vi "Parse TOML String.vi"(8 "error in (no error)":errorcluster, 11 "String":string) -> (0 "error out":errorcluster, 3 "Value":T1)   [LabVIEW 2020, in "TOML.lvlib"]
uses:
  TOML.lvlib
  TOML Value.ctl
  Key-Value Pair.ctl
  Value.ctl
  Value Type.ctl
  State.ctl
  Context.ctl
  Table Context.ctl
  Table Array Context.ctl
  Array Context.ctl
  <vilib>/regexp/Match Regular Expression.xnode
  <vilib>/ErrorRing/Error Ring.xnode
  <vilib>/JDP Science/JDP Science Common Utilities/Timestamp/JDP Timestamp.lvlib
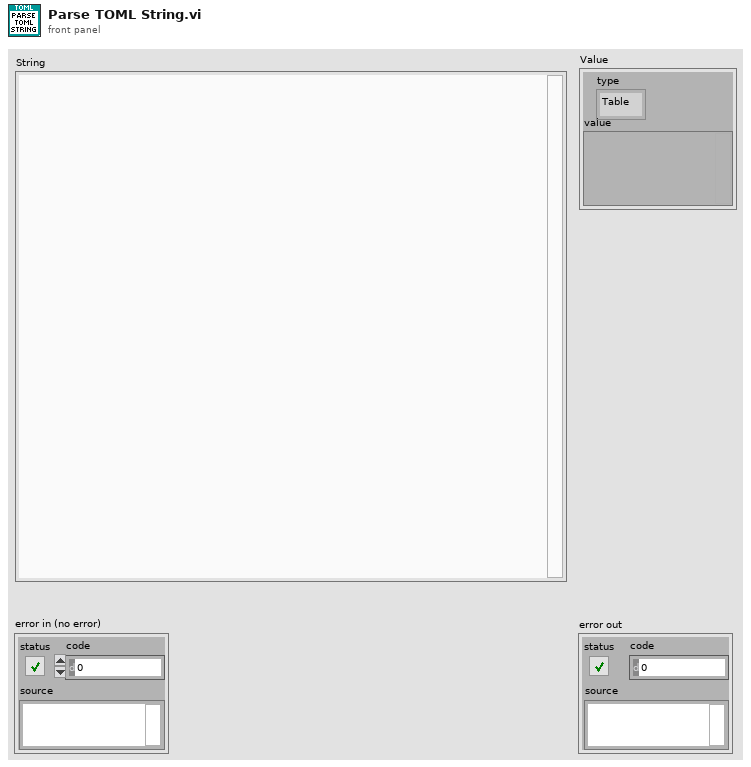
[diagram p1: front panel]
types:
  T1 = typedef "TOML.lvlib/TOML Value.ctl" = cluster{"type":enum16{"Table", "Array", "String", "Integer", "Float", "Boolean", "Offset Date-Time", "Local Date-Time", "Local Date", "Local Time", "Path"}, "value":variant}
  T2 = typedef "TOML.lvlib/Key-Value Pair.ctl" = cluster{"Key":string, "Value":T3}
  T3 = typedef "TOML.lvlib/Value.ctl" = cluster{"Type":T4, "Value":variant}
  T4 = typedef "TOML.lvlib/Value Type.ctl" = enum16{"Table", "Array", "String", "Integer", "Float", "Boolean", "Offset Date-Time", "Local Date-Time", "Local Date", "Local Time", "Path"}
  T5 = enum16{"Table", "Array", "String", "Integer", "Float", "Boolean", "Offset Date-Time", "Local Date-Time", "Local Date", "Local Time"}
  T6 = typedef "TOML.lvlib/Table Context.ctl" = cluster{"Table":T2[], "Key":string, "Defined Keys":string[]}
  T7 = typedef "TOML.lvlib/Context.ctl" = cluster{"Type":enum16{"Table", "Array", "Inline Table", "Table Array"}, "Value":variant}
  T8 = typedef "TOML.lvlib/State.ctl" = enum16{"Table", "Value", "Inline Table"}
  T9 = typedef "TOML.lvlib/Table Array Context.ctl" = cluster{"Table Array":cluster{"Table":T2[]}[], "Index":i32, "Key":string}
  T10 = typedef "TOML.lvlib/Array Context.ctl" = cluster{"Array":T3[], "Index":i32, "Empty":bool, "Type":T4}
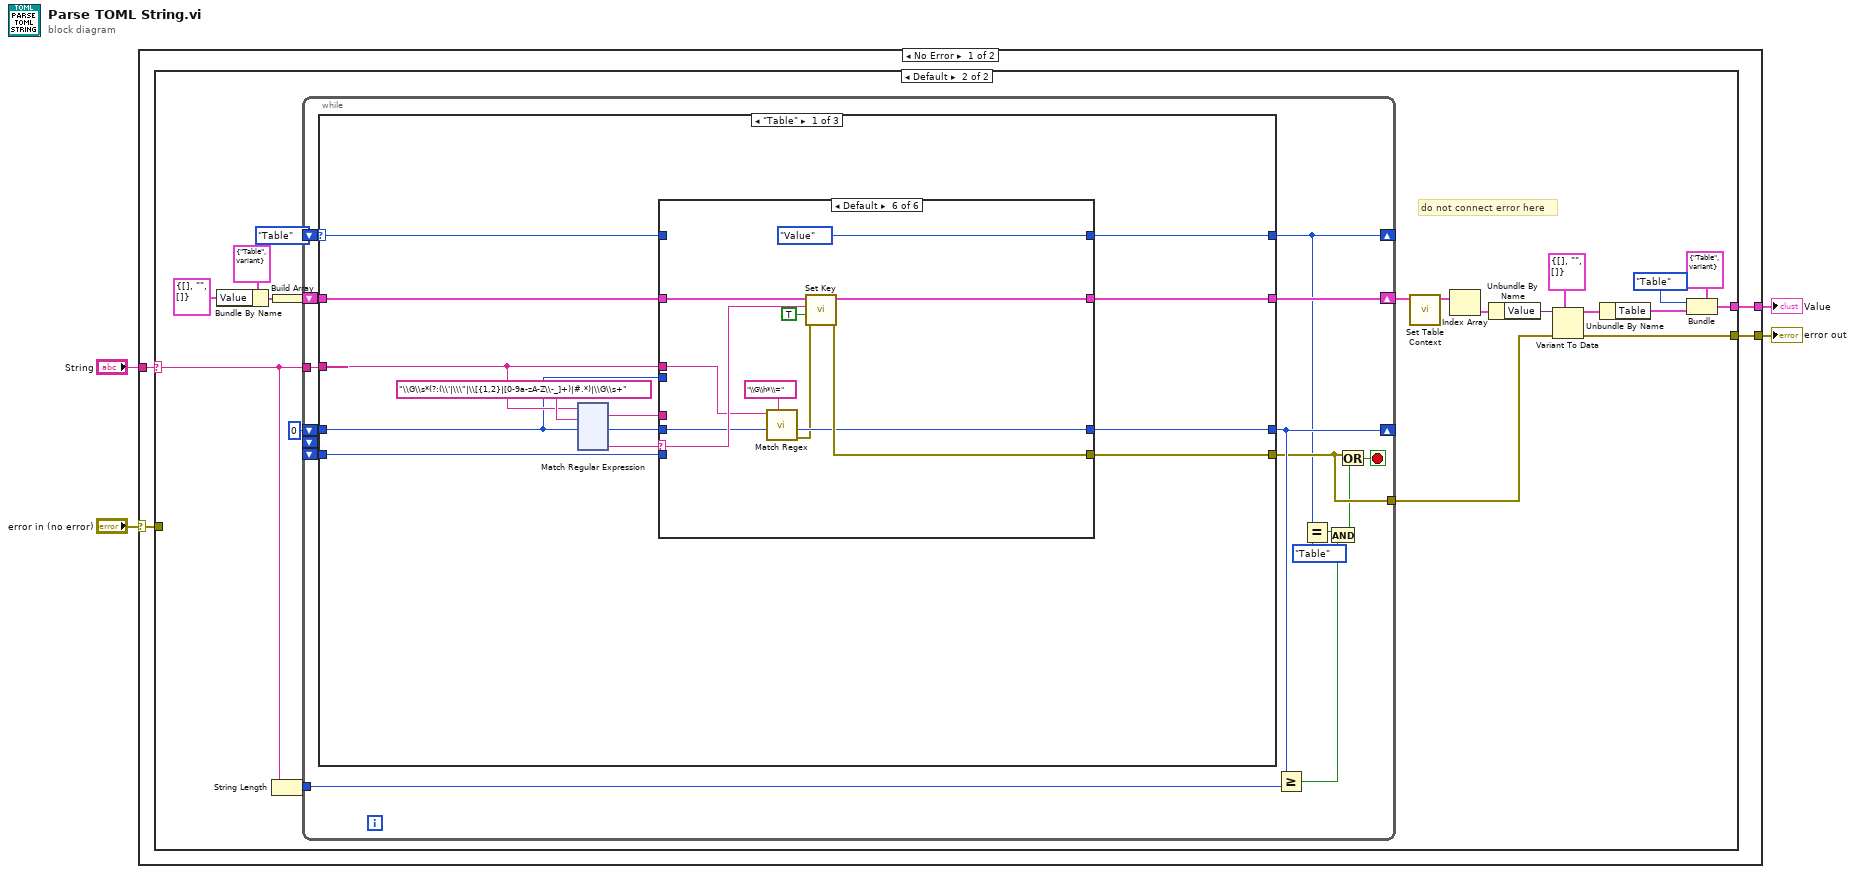
[diagram p0: block diagram]
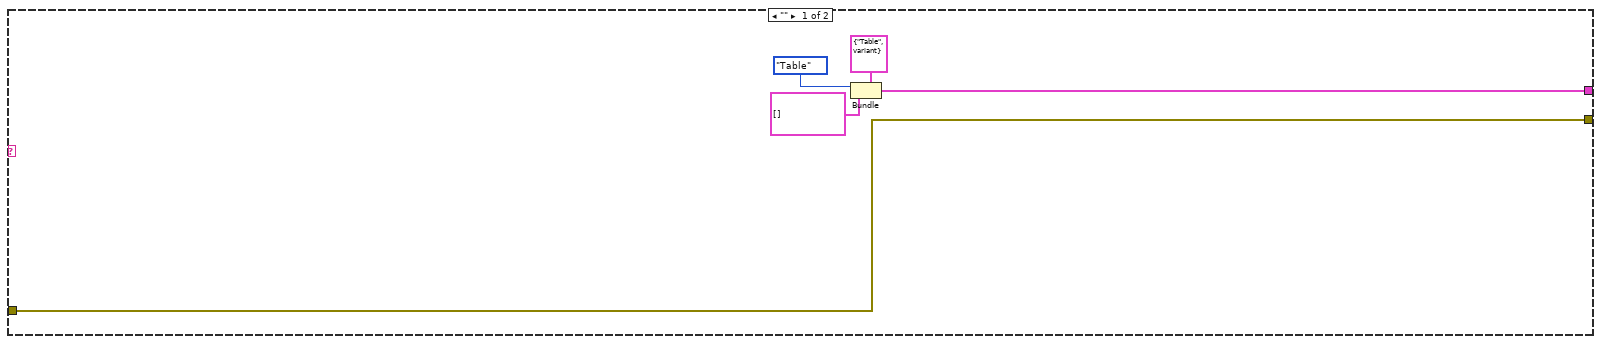
[diagram p2: hidden frame]
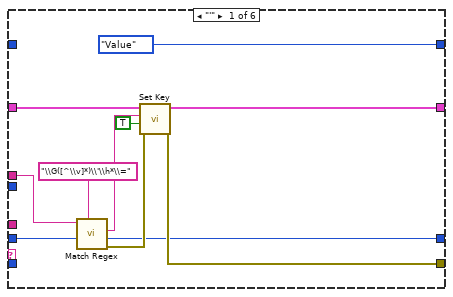
[diagram p3: hidden frame]
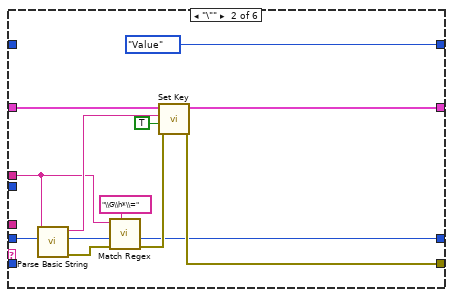
[diagram p4: hidden frame]
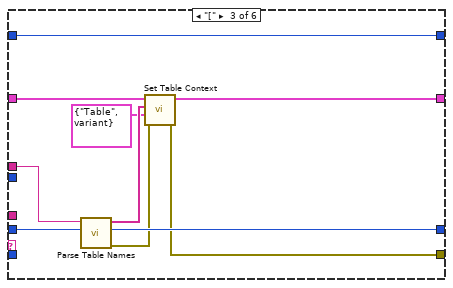
[diagram p5: hidden frame]
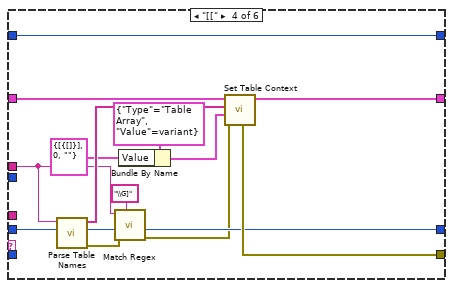
[diagram p6: hidden frame]
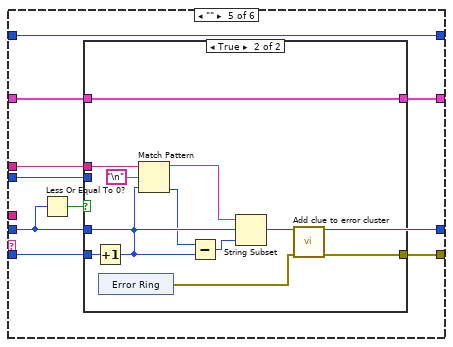
[diagram p7: hidden frame]
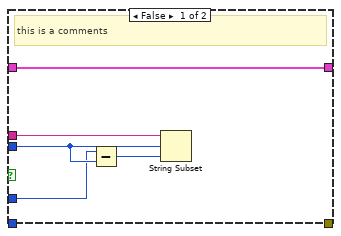
[diagram p8: hidden frame]
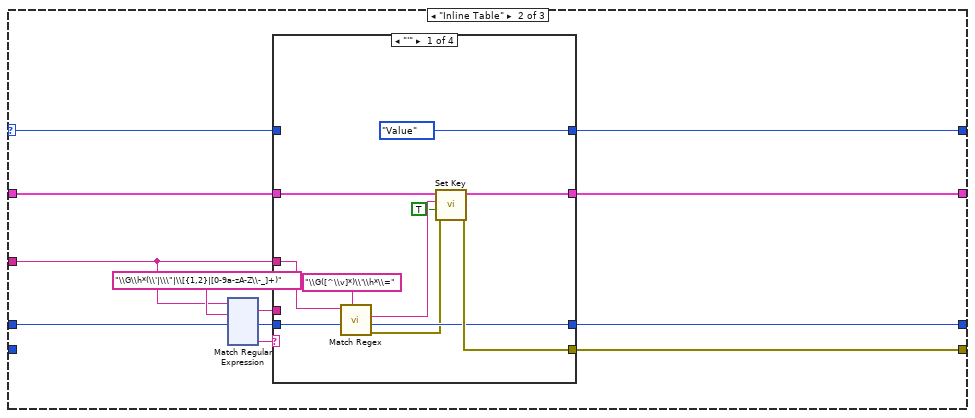
[diagram p9: hidden frame]
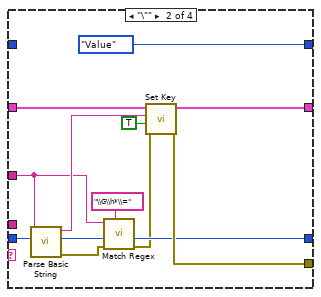
[diagram p10: hidden frame]
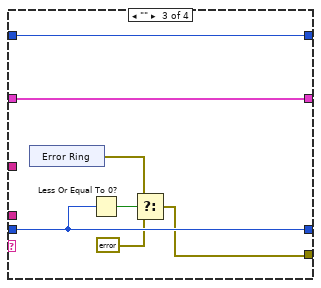
[diagram p11: hidden frame]
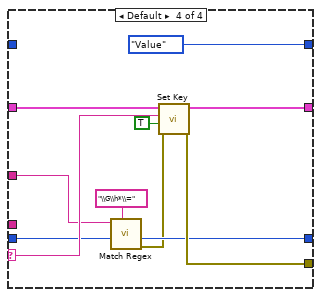
[diagram p12: hidden frame]
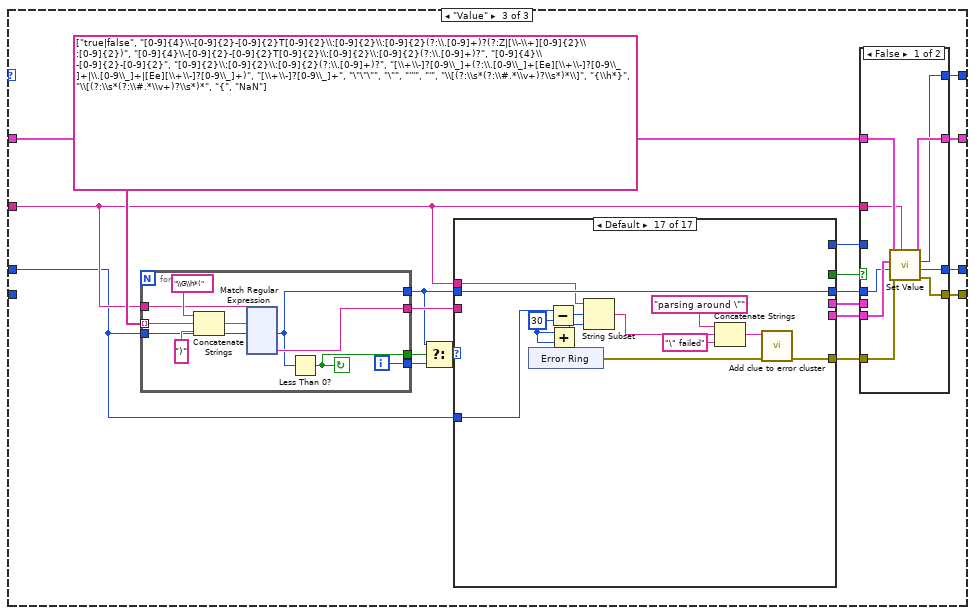
[diagram p13: hidden frame]
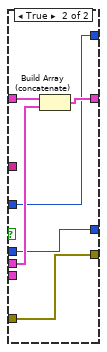
[diagram p14: hidden frame]
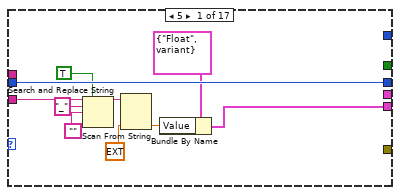
[diagram p15: hidden frame]
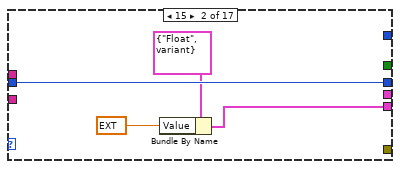
[diagram p16: hidden frame]
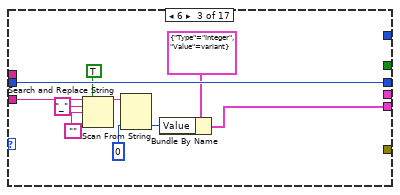
[diagram p17: hidden frame]
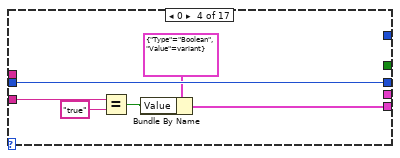
[diagram p18: hidden frame]
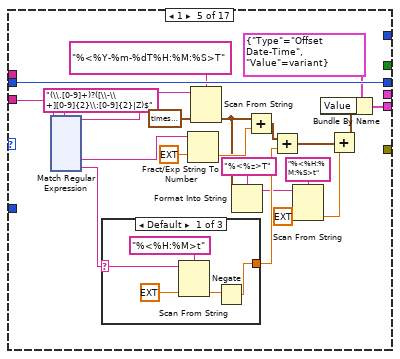
[diagram p19: hidden frame]
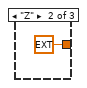
[diagram p20: hidden frame]
diagram:
  n1 = case shown="No Error" "error in (no error)" {
    selector: "error in (no error)" -> [w5 w846]
    tunnel: "String" -> [w8 _]
    tunnel: [w6 _] -> w1
    tunnel: [w7 w846] -> w3
    frame No Error {
      n2 = case shown="Default" w8 {
        selector: w8 -> [_ w32]
        tunnel: [w9 w24] -> w7
        tunnel: [w10 w20] -> w6
        tunnel: w5 -> [w9 _]
        frame "" {
          n3 = Bundle(cluster=T1 {"type"=enum."Table", "value"=variant} ("Value"), "type"=T5."Table" ("Type"), "value"=T2[] [] ("Table")) -> (w10:T1)
        }
        frame Default {
          w15 = 0
          # "do not connect error here"
          n4 = Bundle By Name(cluster=T7 {"Type"=enum."Table", "Value"=variant} ("Context"), "Value"=T6 {"Table"=[], "Key"="", "Defined Keys"=[]} ("Table Context")) -> (w17:T7)
          n5 = String Length(string=w32) -> (length=w31:i32)
          n6 = Build Array(w17) -> (w16:T7[])
          n7 = while {
            tunnel: w32 -> [w47]
            shift-right: [w37] -> _
            shift-left: State."Table" ("State") -> [w48]
            shift-right: [w45] -> w30
            shift-left: w16 -> [w44]
            shift-right: [w40] -> _
            shift-left: w15 -> [w46]
            tunnel: w31 -> [w42]
            tunnel: [w39] -> w14
            shift-left: w15 -> [_]
            shift-left: w15 -> [w34]
            stop <- w43 stop-if-true
            n8 = case shown="\"Table\"" w48 {
              selector: w48 -> [w57 w271 _]
              tunnel: w47 -> [w51 w265 w436]
              tunnel: w46 -> [w49 w264 w435]
              tunnel: [w58 w272 w440] -> w37
              tunnel: [w56 w270 w447] -> w45
              tunnel: w44 -> [w55 w269 w446]
              tunnel: [w59 w273 w437] -> w40
              tunnel: [w54 w268 w444] -> w39
              tunnel: w34 -> [w50 _ _]
              frame "Table" {
                n9 = xnode "Match Regular Expression"("input string"=w51, "regular expression"="\\G\\s*(?:(\\'|\\\"|\\[{1,2}|[0-9a-zA-Z\\-_]+)|#.*)|\\G\\s+", "offset (0)"=w49) -> ("whole match"=w52:string, "offset past match"=w60:i32, "submatch 1"=w53:string)  [unwired: 3 in, 3 out]
                n10 = case shown="Default" w53 {
                  selector: w53 -> [_ _ _ _ _ w143]
                  tunnel: [w63 w74 w92 w101 w113 w139] -> w59
                  tunnel: w60 -> [w64 w85 w93 w109 w113 w140]
                  tunnel: [State."Value" ("State") State."Value" ("State") w95 w110 w119 State."Value" ("State")] -> w58
                  tunnel: w57 -> [_ _ w95 w110 w119 _]
                  tunnel: [w68 w81 w90 w107 w112 w144] -> w56
                  tunnel: w55 -> [w71 w82 w91 w108 w111 w145]
                  tunnel: [w69 w83 w86 w105 w118 w146] -> w54
                  tunnel: w51 -> [w65 w78 w94 w103 w116 w141]
                  tunnel: w52 -> [_ _ _ _ _ _]
                  tunnel: w50 -> [_ _ _ _ w115 _]
                  tunnel: w49 -> [_ _ _ _ w114 _]
                  frame "'" {
                    n11 = call "Match Regex.vi"("regular expression"="\\G([^\\v]*)\\'\\h*\\=", "offset"=w64, "String"=w65) -> ("error out"=w70:errorcluster, "offset past match"=w63:i32, "submatch 1"=w66:string)  [unwired: 5 in, 1 out]
                    n12 = call "Set Key.vi"("error in (no error)"=w70, "Define"=TRUE, "Key"=w66, "Stack in"=w71) -> ("error out"=w69:errorcluster, "Stack out"=w68:T7[])  [unwired: 6 in]
                  }
                  frame "\"" {
                    n13 = call "Parse Basic String.vi"("start at"=w85, "TOML String"=w78) -> ("error out"=w76:errorcluster, "offset past match"=w77:i32, "String"=w80:string)  [unwired: 7 in]
                    n14 = call "Match Regex.vi"("regular expression"="\\G\\h*\\=", "error in (no error)"=w76, "offset"=w77, "String"=w78) -> ("error out"=w75:errorcluster, "offset past match"=w74:i32)  [unwired: 4 in, 2 out]
                    n15 = call "Set Key.vi"("error in (no error)"=w75, "Define"=TRUE, "Key"=w80, "Stack in"=w82) -> ("error out"=w83:errorcluster, "Stack out"=w81:T7[])  [unwired: 6 in]
                  }
                  frame "[" {
                    n16 = call "Parse Table Names.vi"("start at"=w93, "TOML String"=w94) -> ("error out"=w87:errorcluster, "offset past match"=w92:i32, "Table Stack"=w89:string[])  [unwired: 7 in]
                    n17 = call "Set Table Context.vi"("error in (no error)"=w87, "Context"=T7 {"Type"=enum."Table", "Value"=variant}, "Table Names"=w89, "Stack in"=w91) -> ("error out"=w86:errorcluster, "Stack out"=w90:T7[])  [unwired: 6 in]
                  }
                  frame "[[" {
                    n18 = call "Parse Table Names.vi"("start at"=w109, "TOML String"=w103) -> ("error out"=w100:errorcluster, "offset past match"=w102:i32, "Table Stack"=w106:string[])  [unwired: 7 in]
                    n19 = call "Match Regex.vi"("regular expression"="\\G]", "error in (no error)"=w100, "offset"=w102, "String"=w103) -> ("error out"=w99:errorcluster, "offset past match"=w101:i32)  [unwired: 4 in, 2 out]
                    n20 = Bundle By Name(cluster=T7 {"Type"=enum."Table Array", "Value"=variant} ("Context"), "Value"=T9 {"Table Array"=[{"Table"=[]}], "Index"=0, "Key"=""} ("Table Array Context")) -> (w97:T7)
                    n21 = call "Set Table Context.vi"("error in (no error)"=w99, "Context"=w97, "Table Names"=w106, "Stack in"=w108) -> ("error out"=w105:errorcluster, "Stack out"=w107:T7[])  [unwired: 6 in]
                  }
                  frame "" {
                    n22 = Less Or Equal To 0?(x=w113) -> (x <= 0?=w117:bool)
                    n23 = case shown="True" w117 {
                      tunnel: [_ w135] -> w118
                      tunnel: w116 -> [w124 w133]
                      tunnel: w115 -> [_ w131]
                      tunnel: w114 -> [w123 _]
                      tunnel: w113 -> [w122 _]
                      tunnel: [w120 w125] -> w112
                      tunnel: w111 -> [w120 w125]
                      frame False {
                        # "this is a comments"
                        n24 = Subtract(x=w122, y=w123) -> (x-y=w121:i32)
                        n25 = String Subset(string=w124, offset (0)=w123, length (rest)=w121) -> ()  [unwired: 1 out]
                      }
                      frame True {
                        n26 = Increment(x=w131) -> (x+1=w127:i32)
                        n27 = xnode "Error Ring"() -> ("error out"=w134:errorcluster)
                        n28 = Match Pattern(string=w133, regular expression="\n", offset (0)=w127) -> (before substring=w126:string, offset past match=w129:i32)  [unwired: 2 out]
                        n29 = Subtract(x=w129, y=w127) -> (x-y=w130:i32)
                        n30 = String Subset(string=w126, offset (0)=w127, length (rest)=w130) -> (substring=w128:string)
                        n31 = call "Add clue to error cluster.vi"("error in (no error)"=w134, "String"=w128) -> ("error out"=w135:errorcluster)  [unwired: 9 in]
                      }
                    }
                  }
                  frame Default {
                    n32 = call "Match Regex.vi"("regular expression"="\\G\\h*\\=", "offset"=w140, "String"=w141) -> ("error out"=w138:errorcluster, "offset past match"=w139:i32)  [unwired: 5 in, 2 out]
                    n33 = call "Set Key.vi"("error in (no error)"=w138, "Define"=TRUE, "Key"=w143, "Stack in"=w145) -> ("error out"=w146:errorcluster, "Stack out"=w144:T7[])  [unwired: 6 in]
                  }
                }
              }
              frame "Inline Table" {
                n34 = xnode "Match Regular Expression"("input string"=w265, "regular expression"="\\G\\h*(\\'|\\\"|\\[{1,2}|[0-9a-zA-Z\\-_]+)", "offset (0)"=w264) -> ("whole match"=w266:string, "offset past match"=w274:i32, "submatch 1"=w267:string)  [unwired: 3 in, 3 out]
                n35 = case shown="\"'\"" w267 {
                  selector: w267 -> [_ _ _ w314]
                  tunnel: [w279 w292 w305 w310] -> w273
                  tunnel: w274 -> [w280 w299 w305 w311]
                  tunnel: [State."Value" ("State") State."Value" ("State") w301 State."Value" ("State")] -> w272
                  tunnel: w271 -> [_ _ w301 _]
                  tunnel: [w283 w295 w306 w315] -> w270
                  tunnel: w269 -> [w285 w296 w306 w316]
                  tunnel: [w284 w297 w302 w317] -> w268
                  tunnel: w265 -> [w281 w291 _ w312]
                  tunnel: w266 -> [_ _ _ _]
                  frame "'" {
                    n36 = call "Match Regex.vi"("regular expression"="\\G([^\\v]*)\\'\\h*\\=", "offset"=w280, "String"=w281) -> ("error out"=w277:errorcluster, "offset past match"=w279:i32, "submatch 1"=w278:string)  [unwired: 5 in, 1 out]
                    n37 = call "Set Key.vi"("error in (no error)"=w277, "Define"=TRUE, "Key"=w278, "Stack in"=w285) -> ("error out"=w284:errorcluster, "Stack out"=w283:T7[])  [unwired: 6 in]
                  }
                  frame "\"" {
                    n38 = call "Parse Basic String.vi"("start at"=w299, "TOML String"=w291) -> ("error out"=w288:errorcluster, "offset past match"=w293:i32, "String"=w294:string)  [unwired: 7 in]
                    n39 = call "Match Regex.vi"("regular expression"="\\G\\h*\\=", "error in (no error)"=w288, "offset"=w293, "String"=w291) -> ("error out"=w289:errorcluster, "offset past match"=w292:i32)  [unwired: 4 in, 2 out]
                    n40 = call "Set Key.vi"("error in (no error)"=w289, "Define"=TRUE, "Key"=w294, "Stack in"=w296) -> ("error out"=w297:errorcluster, "Stack out"=w295:T7[])  [unwired: 6 in]
                  }
                  frame "" {
                    n41 = xnode "Error Ring"() -> ("error out"=w300:errorcluster)
                    n42 = Less Or Equal To 0?(x=w305) -> (x <= 0?=w304:bool)
                    n43 = Select(t=w300, s=w304, f=errorcluster {"status"=FALSE, "code"=0, "source"=""}) -> (s? t:f=w302:errorcluster)
                  }
                  frame Default {
                    n44 = call "Match Regex.vi"("regular expression"="\\G\\h*\\=", "offset"=w311, "String"=w312) -> ("error out"=w309:errorcluster, "offset past match"=w310:i32)  [unwired: 5 in, 2 out]
                    n45 = call "Set Key.vi"("error in (no error)"=w309, "Define"=TRUE, "Key"=w314, "Stack in"=w316) -> ("error out"=w317:errorcluster, "Stack out"=w315:T7[])  [unwired: 6 in]
                  }
                }
              }
              frame "Value" {
                n46 = for {
                  tunnel: string[] ["true|false", "[0-9]{4}\\-[0-9]{2}-[0-9]{2}T[0-9]{2}\\:[0-9]{2}\\:[0-9]{2}(?:\\.[0-9]+)?(?:Z|[\\-\\+][0-9]{2}\\:[0-9]{2})", "[0-9]{4}\\-[0-9]{2}-[0-9]{2}T[0-9]{2}\\:[0-9]{2}\\:[0-9]{2}(?:\\.[0-9]+)?", "[0-9]{4}\\-[0-9]{2}-[0-9]{2}", "[0-9]{2}\\:[0-9]{2}\\:[0-9]{2}(?:\\.[0-9]+)?", "[\\+\\-]?[0-9\\_]+(?:\\.[0-9\\_]+[Ee][\\+\\-]?[0-9\\_]+|\\.[0-9\\_]+|[Ee][\\+\\-]?[0-9\\_]+)", "[\\+\\-]?[0-9\\_]+", "\"\"\"", "\"", "'''", "'", "\\[(?:\\s*(?:\\#.*\\v+)?\\s*)*\\]", "{\\h*}", "\\[(?:\\s*(?:\\#.*\\v+)?\\s*)*", "{", "NaN"] -> [w729] mode=indexing
                  tunnel: w436 -> [w725]
                  tunnel: w435 -> [w724]
                  tunnel: [w723] -> w449
                  tunnel: [w722] -> w448
                  tunnel: [w721] -> w452
                  tunnel: [w720] -> w451
                  i -> [w720]
                  stop <- w721 continue-if-true
                  n47 = Concatenate Strings("\\G\\h*(" ("string"), w729, ")" ("string")) -> (w726:string)
                  n48 = xnode "Match Regular Expression"("input string"=w725, "regular expression"=w726, "offset (0)"=w724) -> ("offset past match"=w722:i32, "submatch 1"=w723:string)  [unwired: 3 in, 4 out]
                  n49 = Less Than 0?(x=w722) -> (x < 0?=w721:bool)
                }
                n50 = Select(t=w448, s=w452, f=w451) -> (s? t:f=w450:i32)
                n51 = case shown="Default" w450 {
                  tunnel: w449 -> [w473 _ w487 w497 w507 w648 w651 w655 _ _ _ _ _ _ _ _ _]
                  tunnel: w448 -> [w478 w482 w492 w498 w520 w650 w654 w658 w660 w667 w675 w680 w684 w691 w700 w706 w718]
                  tunnel: [w478 w482 w492 w498 w520 w650 w654 w658 w659 w666 w676 w680 w684 w688 w700 w706 w718] -> w438
                  tunnel: [_ _ _ _ _ w647 _ _ _ _ w673 _ _ w687 _ _ w716] -> w445
                  tunnel: [w474 w480 w488 w493 w518 w649 w652 w656 w663 w669 w677 w681 w685 w693 _ _ _] -> w443
                  tunnel: w436 -> [_ _ _ _ _ _ _ _ w662 w668 w672 _ _ w690 _ _ w715]
                  tunnel: [_ _ _ _ _ _ _ _ _ _ _ _ _ _ TRUE TRUE _] -> w442
                  tunnel: [_ _ _ _ _ _ _ _ _ _ _ _ _ _ w696 w703 _] -> w441
                  tunnel: [_ _ _ _ _ _ _ _ _ _ _ _ _ _ State."Value" ("State") State."Inline Table" ("State") _] -> w439
                  tunnel: w435 -> [_ _ _ _ _ _ _ _ _ _ _ _ _ _ _ _ w714]
                  frame 5 {
                    n52 = Search and Replace String(replace all?=TRUE ("replace all? (F)"), input string=w473, search string="_", replace string="") -> (result string=w472:string)  [unwired: 4 in, 3 out]
                    n53 = Scan From String(input string=w472, default 1=ext 0.0 ("default value 1")) -> (output 1=w476:ext)  [unwired: 3 in, 3 out]
                    n54 = Bundle By Name(cluster=T3 {"Type"=enum."Float", "Value"=variant} ("Value"), "Value"=w476) -> (w474:T3)
                  }
                  frame 15 {
                    n55 = Bundle By Name(cluster=T3 {"Type"=enum."Float", "Value"=variant} ("Value"), "Value"=ext nan ("default value 1")) -> (w480:T3)
                  }
                  frame 6 {
                    n56 = Search and Replace String(replace all?=TRUE ("replace all? (F)"), input string=w487, search string="_", replace string="") -> (result string=w486:string)  [unwired: 4 in, 3 out]
                    n57 = Scan From String(input string=w486, default 1=i64 0 ("default value 1")) -> (output 1=w490:i64)  [unwired: 3 in, 3 out]
                    n58 = Bundle By Name(cluster=T3 {"Type"=enum."Integer", "Value"=variant} ("Value"), "Value"=w490) -> (w488:T3)
                  }
                  frame 0 {
                    n59 = Equal?(x=w497, y="true") -> (x = y?=w494:bool)
                    n60 = Bundle By Name(cluster=T3 {"Type"=enum."Boolean", "Value"=variant} ("Value"), "Value"=w494) -> (w493:T3)
                  }
                  frame 1 {
                    n61 = xnode "Match Regular Expression"("input string"=w507, "regular expression"="(\\.[0-9]+)?([\\-\\+][0-9]{2}\\:[0-9]{2}|Z)$") -> ("before match"=w512:string, "submatch 1"=w511:string, "submatch 2"=w509:string)  [unwired: 4 in, 4 out]
                    n62 = case shown="Default" w509 {
                      selector: w509 -> [w525 _ _]
                      tunnel: [w521 ext 0.0 0.0] -> w508
                      frame Default {
                        n63 = Scan From String(format string="%<%H:%M>t", input string=w525, default 1=ext 0.0 ("default value 1")) -> (output 1=w522:ext)  [unwired: 2 in, 3 out]
                        n64 = Negate(x=w522) -> (-x=w521:ext)
                      }
                      frame "Z" {
                      }
                      frame "" {
                      }
                    }
                    n65 = Fract/Exp String To Number(string=w511, default (0 dbl)=ext 0.0 ("default (0 DBL)")) -> (number=w513:ext)  [unwired: 2 in, 1 out]
                    n66 = Scan From String(format string="%<%Y-%m-%dT%H:%M:%S>T", input string=w512, default 1=timestamp(0 s since 1904-01-01)) -> (output 1=w499:timestamp)  [unwired: 2 in, 3 out]
                    n67 = Format Into String(format string="%<%z>T", w499) -> (resulting string=w502:string)  [unwired: 2 in, 1 out]
                    n68 = Add(x=w499, y=w513) -> (x+y=w510:timestamp)
                    n69 = Add(x=w510, y=w508) -> (x+y=w506:timestamp)
                    n70 = Scan From String(format string="%<%H:%M:%S>t", input string=w502, default 1=ext 0.0 ("default value 1")) -> (output 1=w501:ext)  [unwired: 2 in, 3 out]
                    n71 = Add(x=w506, y=w501) -> (x+y=w500:timestamp)
                    n72 = Bundle By Name(cluster=T3 {"Type"=enum."Offset Date-Time", "Value"=variant} ("Value"), "Value"=w500) -> (w518:T3)
                  }
                  frame 2 {
                    n73 = call <vilib>:"Text to Timestamp.vi"("Text Timestamp"=w648) -> ("error out"=w647:errorcluster, "Time Stamp"=w645:timestamp)  [unwired: 7 in, 2 out]
                    n74 = Bundle By Name(cluster=T3 {"Type"=enum."Local Date-Time", "Value"=variant} ("Value"), "Value"=w645) -> (w649:T3)
                  }
                  frame 3 {
                    n75 = Bundle By Name(cluster=T3 {"Type"=enum."Local Date", "Value"=variant} ("Value"), "Value"=w651) -> (w652:T3)
                  }
                  frame 4 {
                    n76 = Bundle By Name(cluster=T3 {"Type"=enum."Local Time", "Value"=variant} ("Value"), "Value"=w655) -> (w656:T3)
                  }
                  frame 7 {
                    n77 = call "Parse Multiline Basic String.vi"("start at"=w660, "TOML String"=w662) -> ("offset past match"=w659:i32, "String"=w661:string)  [unwired: 7 in, 1 out]
                    n78 = Bundle By Name(cluster=T3 {"Type"=enum."String", "Value"=variant} ("Value"), "Value"=w661) -> (w663:T3)
                  }
                  frame 8 {
                    n79 = call "Parse Basic String.vi"("start at"=w667, "TOML String"=w668) -> ("offset past match"=w666:i32, "String"=w665:string)  [unwired: 7 in, 1 out]
                    n80 = Bundle By Name(cluster=T3 {"Type"=enum."String", "Value"=variant} ("Value"), "Value"=w665) -> (w669:T3)
                  }
                  frame 10 {
                    n81 = call "Match Regex.vi"("regular expression"="\\G([^\\v]*)\\'", "offset"=w675, "String"=w672) -> ("error out"=w673:errorcluster, "offset past match"=w676:i32, "submatch 1"=w674:string)  [unwired: 5 in, 1 out]
                    n82 = Bundle By Name(cluster=T3 {"Type"=enum."String", "Value"=variant} ("Value"), "Value"=w674) -> (w677:T3)
                  }
                  frame 11 {
                    n83 = Bundle By Name(cluster=T3 {"Type"=enum."Array", "Value"=variant} ("Value"), "Value"=T3[] []) -> (w681:T3)
                  }
                  frame 12 {
                    n84 = Bundle By Name(cluster=T3 {"Type"=enum."Table", "Value"=variant} ("Value"), "Value"=T2[] []) -> (w685:T3)
                  }
                  frame 9 {
                    n85 = call "Match Regex.vi"("regular expression"="\\G(?:\\r\\h*|\\n\\h*|\\r\\n\\h*)?((?s:.)*?)'''", "offset"=w691, "String"=w690) -> ("error out"=w687:errorcluster, "offset past match"=w688:i32, "submatch 1"=w692:string)  [unwired: 5 in, 1 out]
                    n86 = Bundle By Name(cluster=T3 {"Type"=enum."String", "Value"=variant} ("Value"), "Value"=w692) -> (w693:T3)
                  }
                  frame 13 {
                    n87 = Bundle By Name(cluster=T7 {"Type"=enum."Array", "Value"=variant} ("Context"), "Value"=T10 {"Array"=[], "Index"=0, "Empty"=TRUE, "Type"=enum."Table"} ("Array Context")) -> (w696:T7)
                  }
                  frame 14 {
                    n88 = Bundle By Name(cluster=T7 {"Type"=enum."Inline Table", "Value"=variant} ("Context"), "Value"=T6 {"Table"=[], "Key"="", "Defined Keys"=[]} ("Table Context")) -> (w703:T7)
                  }
                  frame Default {
                    w711 = 30 ("y")
                    n89 = xnode "Error Ring"() -> ("error out"=w717:errorcluster)
                    n90 = Subtract(x=w714, y=w711) -> (x-y=w713:i32)
                    n91 = Add(x=w711, y=w711) -> (x+y=w712:i32)
                    n92 = String Subset(string=w715, offset (0)=w713, length (rest)=w712) -> (substring=w710:string)
                    n93 = Concatenate Strings("parsing around \"" ("string"), w710, "\" failed" ("string")) -> (w709:string)
                    n94 = call "Add clue to error cluster.vi"("error in (no error)"=w717, "String"=w709) -> ("error out"=w716:errorcluster)  [unwired: 9 in]
                  }
                }
                n95 = case shown="False" w442 {
                  tunnel: [w462 w466] -> w447
                  tunnel: w446 -> [w461 w467]
                  tunnel: w445 -> [w460 w468]
                  tunnel: [w459 w468] -> w444
                  tunnel: w443 -> [w458 _]
                  tunnel: w441 -> [_ w465]
                  tunnel: [w457 w464] -> w440
                  tunnel: w439 -> [_ w464]
                  tunnel: w438 -> [w456 w463]
                  tunnel: [w455 w463] -> w437
                  tunnel: w436 -> [w454 _]
                  frame False {
                    n96 = call "Set Value.vi"("TOML string"=w454, "error in (no error)"=w460, "start position"=w456, "Value"=w458, "Context in"=w461) -> ("error out"=w459:errorcluster, "offset past match"=w455:i32, "State"=w457:T8, "Context out"=w462:T7[])  [unwired: 3 in]
                  }
                  frame True {
                    n97 = Build Array (concatenate)(w467, w465) -> (w466:T7[])
                  }
                }
              }
            }
            n98 = Greater Or Equal?(x=w40, y=w42) -> (x >= y?=w41:bool)
            n99 = Equal?(x=w37, y=State."Table") -> (x = y?=w35:bool)
            n100 = And(x=w35, y=w41) -> (x .and. y?=w38:bool)
            n101 = Or(x=w39, y=w38) -> (x .or. y?=w43:bool)
          }
          n102 = call "Set Table Context.vi"("Stack in"=w30) -> ("Stack out"=w29:T7[])  [unwired: 9 in, 1 out]
          n103 = Index Array(array=w29) -> (element=w27:T7)  [unwired: 1 in]
          n104 = Unbundle By Name(w27) -> ("Value"=w26:variant)
          n105 = Variant To Data(error in=w14, type=T6 {"Table"=[], "Key"="", "Defined Keys"=[]} ("Table Context"), Variant=w26) -> (data=w25:T6, error out=w24:errorcluster)
          n106 = Unbundle By Name(w25) -> ("Table"=w21:T2[])
          n107 = Bundle(cluster=T1 {"type"=enum."Table", "value"=variant} ("Value"), "type"=T5."Table" ("Type"), "value"=w21) -> (w20:T1)
        }
      }
    }
    frame Error {
    }
  }
  "error out" <- w3
  "Value" <- w1
